vi "Close Generic Object Refnum (Array VI)__ogtk.vi"(8 "error in (no error)":errorcluster, 9 "timeout in ms (-1)":i32=-1, 10 "wait on unloaded? (FALSE)":bool, 11 "Gen Refnum Array":refnum<vi>[](array[refnum])) -> (0 "error out":errorcluster, 2 "timed out?":bool)   [LabVIEW 2017]
panel:
  # "Close Generic Object Refnum.vi\n\nThis VI is polymorphic to allow closing an array of refnums.\n\nPlease visit http://www.OpenG.org to learn about the\nOpen Source LabVIEW software movement.\n\nNOTICE -- YOU MUST LEAVE THIS NOTICE IN PLACE.  PER THE TERMS OF THE LICENSE BELOW, YOU MAY SUBLICENSE THIS SOFTWARE \nIN ANY WAY THAT DOES NOT CONFLICT WITH THIS LICENSE.\n\n### BSD License (http://www.opensource.org/licenses/bsd-license.php) Begin ###\n \nCopyright (c) 2002, Jim Kring <jim@jimkring.com>\nCopyright (c) 2002, Cal-Bay Systems, Inc. <info@calbay.com>\n\nAll rights reserved.\n\nRedistribution and use in source and binary forms, with or without modification, are permitted provided that the following conditions are met:\n\n    * Redistributions of source code must retain the above copyright notice, this list of conditions and the following disclaimer.\n    * Redistributions in binary form must reproduce the above copyright notice, this list of conditions and the following disclaimer in the \n       documentation and/or other materials provided with the distribution.\n    * Neither the name of SciWare, James Kring, Inc., nor the names of its contributors may be used to endorse or promote products derived \n       from this software without specific prior written permission.\n\nTHIS SOFTWARE IS PROVIDED BY THE COPYRIGHT HOLDERS AND CONTRIBUTORS \"AS IS\" AND ANY EXPRESS OR IMPLIED WARRANTIES, \nINCLUDING, BUT NOT LIMITED TO, THE IMPLIED WARRANTIES OF MERCHANTABILITY AND FITNESS FOR A PARTICULAR PURPOSE ARE \nDISCLAIMED. IN NO EVENT SHALL THE COPYRIGHT OWNER OR CONTRIBUTORS BE LIABLE FOR ANY DIRECT, INDIRECT, INCIDENTAL,\n SPECIAL, EXEMPLARY, OR CONSEQUENTIAL DAMAGES (INCLUDING, BUT NOT LIMITED TO, PROCUREMENT OF SUBSTITUTE GOODS OR \nSERVICES; LOSS OF USE, DATA, OR PROFITS; OR BUSINESS INTERRUPTION) HOWEVER CAUSED AND ON ANY THEORY OF LIABILITY, \nWHETHER IN CONTRACT, STRICT LIABILITY, OR TORT (INCLUDING NEGLIGENCE OR OTHERWISE) ARISING IN ANY WAY OUT OF THE USE \nOF THIS SOFTWARE, EVEN IF ADVISED OF THE POSSIBILITY OF SUCH DAMAGE.\n\n### BSD License End ###"
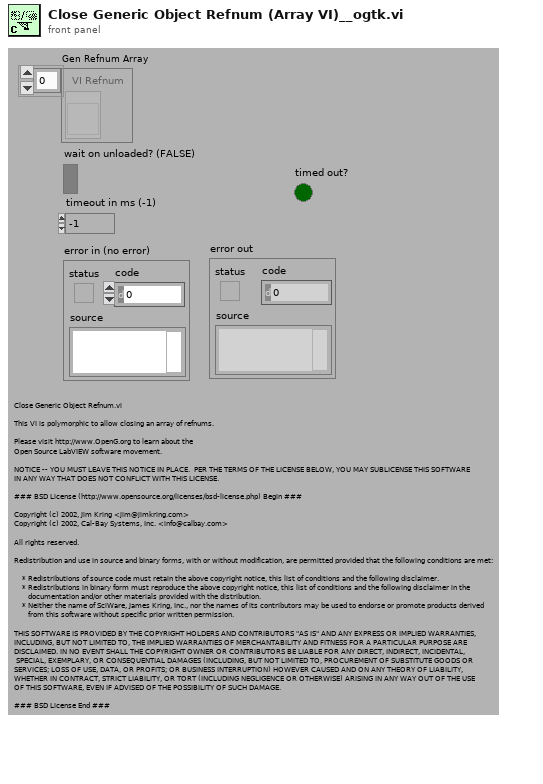
[diagram p1: front panel]
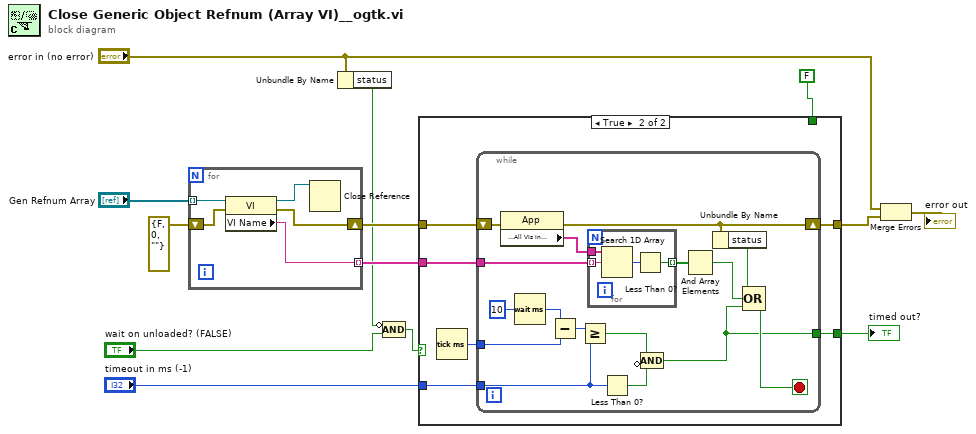
[diagram p0: block diagram]
diagram:
  n1 = for {
    tunnel: "Gen Refnum Array" -> [w18] mode=indexing
    tunnel: [w16] -> w7 mode=indexing
    shift-right: [w14] -> w6
    shift-left: errorcluster {"status"=FALSE, "code"=0, "source"=""} ("error out") -> [w15]
    n2 = property class="VI"(reference=w18, error in=w15) -> (reference out=w17:refnum<vi>, error out=w14:errorcluster, "VI Name"=w16:string)
    n3 = Close Reference(reference=w17) -> ()  [unwired: 1 in, 1 out]
  }
  n4 = Unbundle By Name("error in (no error)") -> ("status"=w1:bool)
  n5 = Compound Arithmetic op=AND(invert w1, "wait on unloaded? (FALSE)") -> (w4:bool)
  n6 = case shown="True" w4 {
    tunnel: w6 -> [w20 w26]
    tunnel: w7 -> [_ w25]
    tunnel: [w19 w23] -> w12
    tunnel: [w20 w22] -> w8
    tunnel: "timeout in ms (-1)" -> [_ w21]
    tunnel: FALSE -> [w19 _]
    frame False {
    }
    frame True {
      n7 = Tick Count (ms)() -> (millisecond timer value=w24:u32)
      n8 = while {
        tunnel: [w27] -> w23
        tunnel: w21 -> [w30]
        tunnel: w24 -> [w37]
        tunnel: w25 -> [w40]
        shift-left: w26 -> [w42]
        shift-right: [w35] -> w22
        stop <- w32 stop-if-true
        n9 = property class="App"(error in=w42) -> (error out=w35:errorcluster, "Application:All VIs In Memory"=w41:string[])  [unwired: 1 in, 1 out]
        n10 = Wait (ms)(milliseconds to wait=u32 10) -> (millisecond timer value=w38:u32)
        n11 = Subtract(x=w38, y=w37) -> (x-y=w36:u32)
        n12 = Greater Or Equal?(x=w36, y=w30) -> (x >= y?=w28:bool)
        n13 = for {
          tunnel: w41 -> [w46]
          tunnel: w40 -> [w45] mode=indexing
          tunnel: [w43] -> w33 mode=indexing
          n14 = Search 1D Array(1D array=w46, element=w45) -> (index of element=w44:i32)  [unwired: 1 in]
          n15 = Less Than 0?(x=w44) -> (x < 0?=w43:bool)
        }
        n16 = Less Than 0?(x=w30) -> (x < 0?=w29:bool)
        n17 = Compound Arithmetic op=AND(w28, invert w29) -> (w27:bool)
        n18 = And Array Elements(Boolean array=w33) -> (logical AND=w31:bool)
        n19 = Unbundle By Name(w35) -> ("status"=w34:bool)
        n20 = Compound Arithmetic op=OR(w34, w31, w27) -> (w32:bool)
      }
    }
  }
  "timed out?" <- w12
  n21 = Merge Errors("error in (no error)", w8) -> (→"error out":errorcluster)
